vi "Factory.vi"(8 "error in (no error)":errorcluster, 11 "File Parsing Interface in":refnum<class "File Parsing Interface.lvclass">) -> (0 "error out":errorcluster, 3 "File Parsing Interface out":refnum<class "File Parsing Interface.lvclass">)   [LabVIEW 2018, in "File Parsing Interface.lvlib" / "File Parsing Interface.lvclass"]
uses:
  File Parsing Interface.lvclass
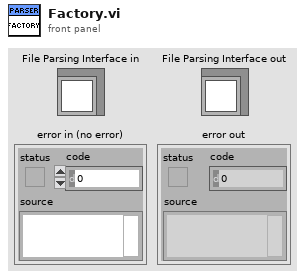
[diagram p1: front panel]
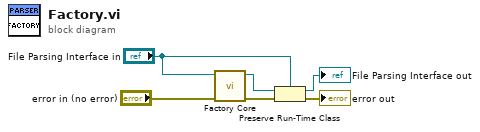
[diagram p0: block diagram]
diagram:
  n1 = call-dynamic "Factory Core.vi"("error in (no error)"="error in (no error)", "Factory Plugin Framework in"="File Parsing Interface in") -> ("error out"=w5:errorcluster, "Factory Plugin Framework out"=w6:refnum<class "File Parsing Interface.lvclass">)  [unwired: 8 in]
  n2 = Preserve Run-Time Class(object in=w6, error in=w5, 2:"File Parsing Interface in") -> (object out=→"File Parsing Interface out":refnum<class "File Parsing Interface.lvclass">, error out=→"error out":errorcluster)
